vi "SeCrTs-Pumb RT Connected.vi"(7 "Enum":enum16{"Read", "Write"}(ring), 8 "error in":errorcluster, 10 "Pumb rt con":bool) -> (0 "error out":errorcluster, 2 "Pumb rt con R":bool)   [LabVIEW 2022 SP3]
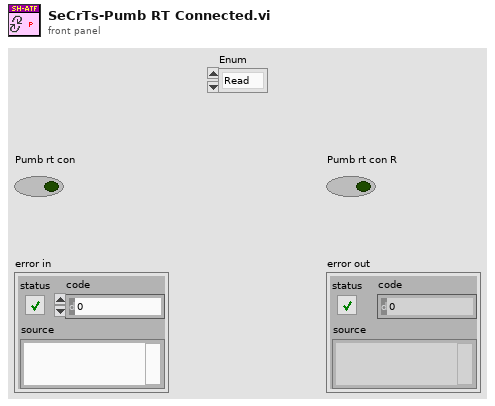
[diagram p1: front panel]
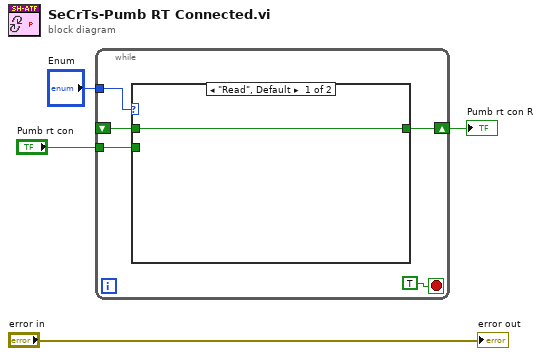
[diagram p0: block diagram]
diagram:
  n1 = while {
    tunnel: "Enum" -> [w9]
    tunnel: "Pumb rt con" -> [w6]
    shift-right: [w7] -> w2
    shift-left: _ -> [w5]
    stop <- TRUE stop-if-true
    n2 = case shown="\"Read\", Default" w9 {
      tunnel: [w10 w11] -> w7
      tunnel: w6 -> [_ w11]
      tunnel: w5 -> [w10 _]
      frame "Read", Default {
      }
      frame "Write" {
      }
    }
  }
  "Pumb rt con R" <- w2
  "error out" <- "error in"
